vi "旋转矩形（TB）.vi"(11 "矩形":T1) -> (3 "旋转后矩形（90）":T1)   [LabVIEW 2011]
uses:
  RectTB.ctl
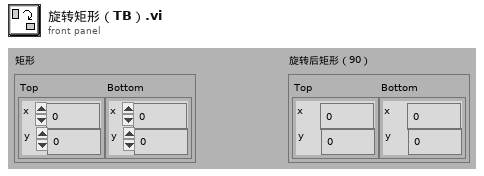
[diagram p1: front panel]
types:
  T1 = typedef "RectTB.ctl" = cluster{"Top":cluster{"x":i16, "y":i16}, "Bottom":cluster{"x":i16, "y":i16}}
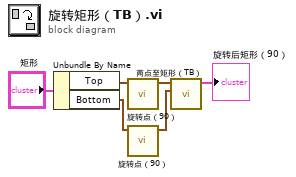
[diagram p0: block diagram]
diagram:
  n1 = Unbundle By Name("矩形") -> ("Top"=w6:cluster{"x":i16, "y":i16}, "Bottom"=w5:cluster{"x":i16, "y":i16})
  n2 = call "旋转点（90）.vi"("点"=w6) -> ("点（90旋转）"=w3:cluster{"x":i16, "y":i16})  [unwired: 10 in]
  n3 = call "旋转点（90）.vi"("点"=w5) -> ("点（90旋转）"=w2:cluster{"x":i16, "y":i16})  [unwired: 10 in]
  n4 = call "两点至矩形（TB）.vi"("point b"=w2, "point a"=w3) -> ("RectTB"=→"旋转后矩形（90）":T1)  [unwired: 9 in]
